vi "Flock_Shared_Wait for Close.vi"(8 "error in (no error)":errorcluster) -> (0 "error out":errorcluster)   [LabVIEW 2013, in "Flock_Shared_Messaging.lvlib" / "Flock_Shared_CentralProcessMessaging.lvlib"]
uses:
  Flock_Shared_CentralProcessMessaging.lvlib
  Flock_Shared_Messaging.lvlib
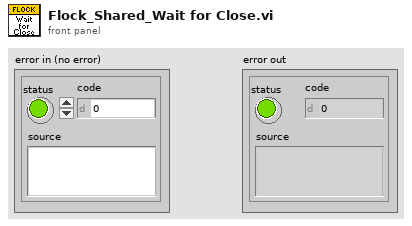
[diagram p1: front panel]
types:
  T1 = typedef "Flock_Shared_Messaging.lvlib/FGV_Queues.ctl" = cluster{"Local Queue in 2":T2, "Enum":T3}[]
  T2 = typedef "amc_Message Queue.ctl" = refnum<queue>
  T3 = typedef "Flock_Shared_Messaging.lvlib/ProcessList.ctl" = string
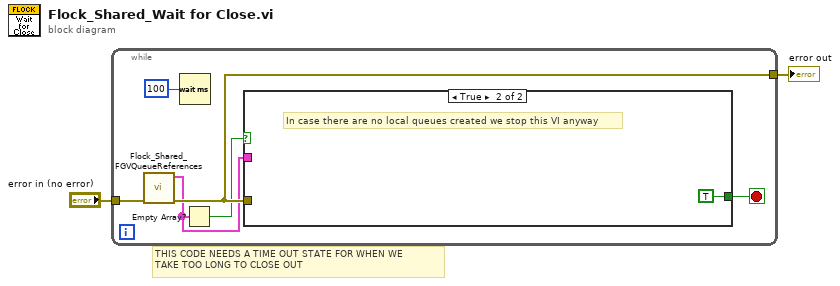
[diagram p0: block diagram]
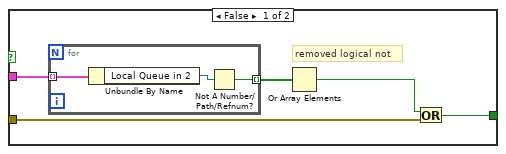
[diagram p2: hidden frame]
diagram:
  # "THIS CODE NEEDS A TIME OUT STATE FOR WHEN WE \nTAKE TOO LONG TO CLOSE OUT"
  n1 = while {
    tunnel: "error in (no error)" -> [w7]
    tunnel: [w6] -> w1
    stop <- w8 stop-if-true
    n2 = call "Flock_Shared_FGVQueueReferences.vi"("error in (no error)"=w7) -> ("error out"=w6:errorcluster, "Array"=w5:T1)  [unwired: 8 in, 1 out]
    n3 = Wait (ms)(milliseconds to wait=u32 100) -> ()  [unwired: 1 out]
    n4 = Empty Array?(array=w5) -> (empty?=w4:bool)
    n5 = case shown="True" w4 {
      tunnel: [w13 TRUE] -> w8
      tunnel: w6 -> [w12 _]
      tunnel: w5 -> [w11 _]
      frame False {
        # "removed logical not"
        n6 = for {
          tunnel: w11 -> [w16] mode=indexing
          tunnel: [w14] -> w10 mode=indexing
          n7 = Unbundle By Name(w16) -> ("Local Queue in 2"=w15:T2)
          n8 = Not A Number/Path/Refnum?(number/path/refnum=w15) -> (NaN/Path/Refnum?=w14:bool)
        }
        n9 = Or Array Elements(Boolean array=w10) -> (logical OR=w9:bool)
        n10 = Or(x=w9, y=w12) -> (x .or. y?=w13:bool)
      }
      frame True {
        # "In case there are no local queues created we stop this VI anyway"
      }
    }
  }
  "error out" <- w1
